vi "Cobra_Serial_Test.vi"() -> ()   [LabVIEW 2015]
panel:
  out "Parsed command string sent to device":string
  in  "Send Data Button":bool
  in  "Configuration string to device":string
  out "Characters Read":u32
  out "IMAQ Session Out":refnum<k11>
  out "Returned string from device":string
  out "error out":errorcluster
  in  "error in (no error)":errorcluster
  # "Introduction:\n  This project serves as a basic example on how to send configuration\n   strings to a WP Cobra OCT Spectrometer. \n\nInstructions:\n  1. Run VI\n  2. Enter configuration string in text box to the left\n  3. Hit the send button\n  4. Returned information will be displayed"
  # "Serial protocol documentation:\n  http://wasatchdevices.com/cobra-camera-link-commands/"
  # "Note:\n  You will not be able to view output spectra in \n  NI MAX while this project is running."
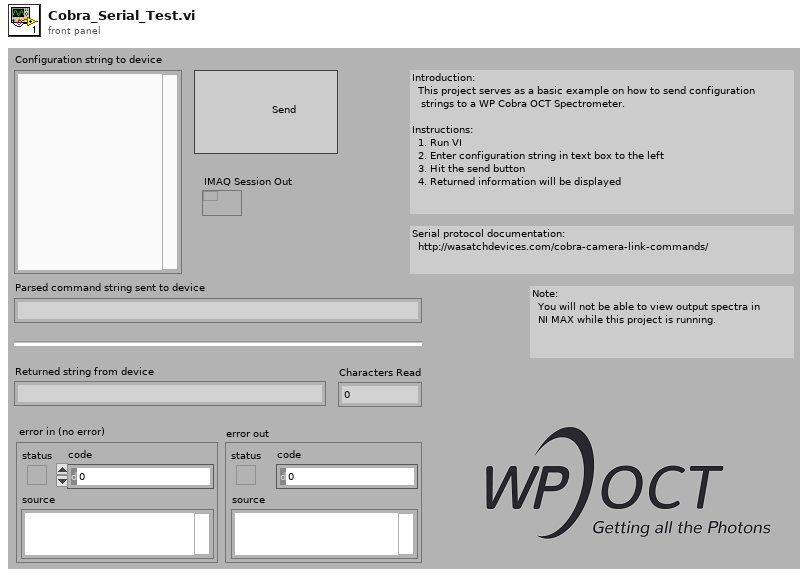
[diagram p1: front panel]
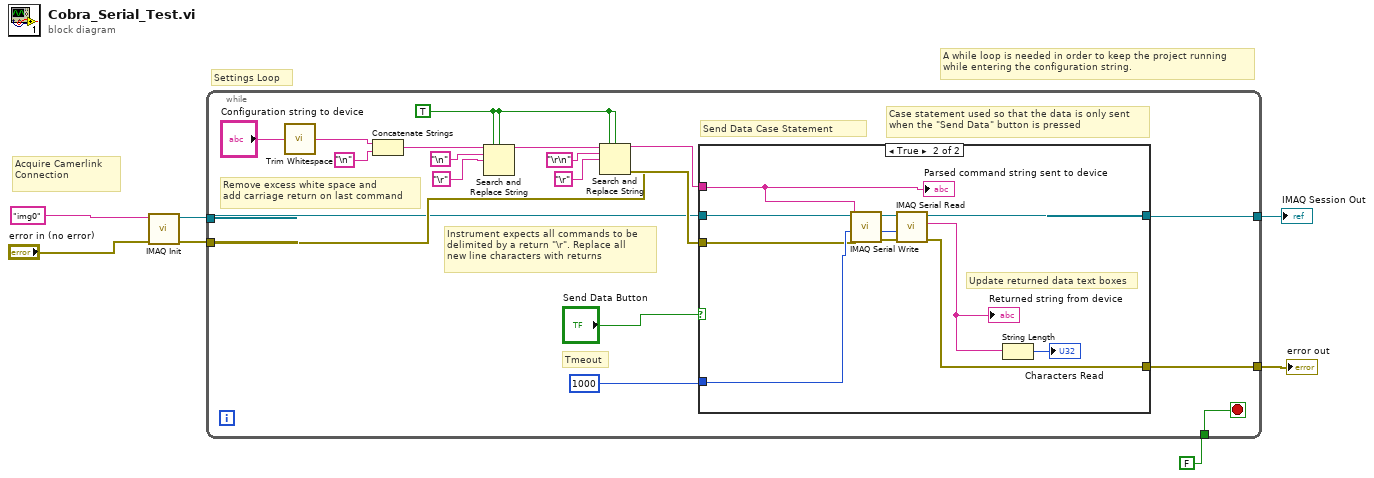
[diagram p0: block diagram]
diagram:
  # "Acquire Camerlink Connection"
  # "A while loop is needed in order to keep the project running\nwhile entering the configuration string."
  # "Settings Loop"
  n1 = call <vilib>:"IMAQ Init.vi"("error in (no error)"="error in (no error)", "Interface Name"="img0") -> ("error out"=w4:errorcluster, "IMAQ Session Out"=w3:refnum<k11>)  [unwired: 8 in]
  n2 = while {
    tunnel: [w25] -> w5
    tunnel: w4 -> [w18]
    tunnel: w3 -> [w8]
    tunnel: [w24] -> w2
    tunnel: FALSE -> [w22]
    stop <- w22 stop-if-true
    w11 = TRUE
    # "Send Data Case Statement"
    # "Instrument expects all commands to be\ndelimited by a return \"\\r\". Replace all \nnew line characters with returns"
    # "Remove excess white space and \nadd carriage return on last command"
    # "Case statement used so that the data is only sent \nwhen the \"Send Data\" button is pressed"
    # "Tmeout"
    n3 = call <vilib>:"Trim Whitespace.vi"("string"="Configuration string to device") -> ("trimmed string"=w14:string)  [unwired: 1 in]
    n4 = Concatenate Strings(w14, "\n") -> (w13:string)
    n5 = Search and Replace String(replace all?=w11, case sensitive?=w11, input string=w13, search string="\n", replace string="\r") -> (result string=w17:string)  [unwired: 3 in, 3 out]
    n6 = Search and Replace String(replace all?=w11, case sensitive?=w11, input string=w17, search string="\r\n", replace string="\r", error in=w18) -> (result string=w16:string, error out=w20:errorcluster)  [unwired: 2 in, 2 out]
    n7 = case shown="True" "Send Data Button" {
      tunnel: 1000 -> [_ w36]
      tunnel: [w28 w35] -> w25
      tunnel: w20 -> [w28 w30]
      tunnel: [w27 w34] -> w24
      tunnel: w16 -> [_ w31]
      tunnel: w8 -> [w27 w29]
      frame False {
      }
      frame True {
        # "Update returned data text boxes"
        n8 = call <vilib>:"IMAQ Serial Write.vi"("error in (no error)"=w30, "Timeout"=w36, "String to write"=w31, "IMAQ Session In"=w29) -> ("error out"=w38:errorcluster, "IMAQ Session Out"=w37:refnum<k11>)  [unwired: 4 in]
        n9 = call <vilib>:"IMAQ Serial Read.vi"("error in (no error)"=w38, "Timeout"=w36, "IMAQ Session In"=w37) -> ("error out"=w35:errorcluster, "String Read"=w33:string, "IMAQ Session Out"=w34:refnum<k11>)  [unwired: 3 in, 1 out]
        "Returned string from device" <- w33
        n10 = String Length(string=w33) -> (length=→"Characters Read":i32)
        "Parsed command string sent to device" <- w31
      }
    }
  }
  "error out" <- w5
  "IMAQ Session Out" <- w2
